vi "Test.vi"() -> ()   [LabVIEW 2014]
uses:
  <vilib>/Utility/file.llb/Read From Spreadsheet File (DBL).vi
  <vilib>/imath/engines/lvmath2/RunTimeEngine/ArithmeticOperatorToken/NIMS_ArithmeticOperator_minus.vi
  <instcachedir>/0/NIMS_ArithmeticOperator_minus_39C0593E74DA4138ACA2AB742906488D.lvgen/NIMS_ArithmeticOperator_minus_39C0593E74DA4138ACA2AB742906488D_003.vi
  <vilib>/imathl/engines/lvmath/Functions/Error Handling/Create Error.vi
  <vilib>/imath/engines/lvmath2/RunTimeEngine/NodeEndStatement/NIMS_NodeEndStatement_Output.vi
  <instcachedir>/0/NIMS_NodeEndStatement_Output_53EC0D466D134D7ABD903AC30B43404B.lvgen/NIMS_NodeEndStatement_Output_53EC0D466D134D7ABD903AC30B43404B_005.vi
  <vilib>/imath/engines/lvmath2/RunTimeEngine/ErrorHandling/NIMS_Finalize Error.vi
panel:
  out "new points":dbl[][](array[numeric]) format="%0.3f"
  out "Local coordinates":dbl[][](array[numeric]) format="%0.3f"
  out "Ynew":dbl[](array[numeric])
  out "Xnew":dbl[](array[numeric])
  in  "File path for new point":path
  in  "File path for local coordinates":path
  in  "File path for global coordinates":path
  out "Global coordinates":dbl[][](array[numeric]) format="%0.3f"
  out "resY":dbl[](array[numeric])
  out "resX":dbl[](array[numeric])
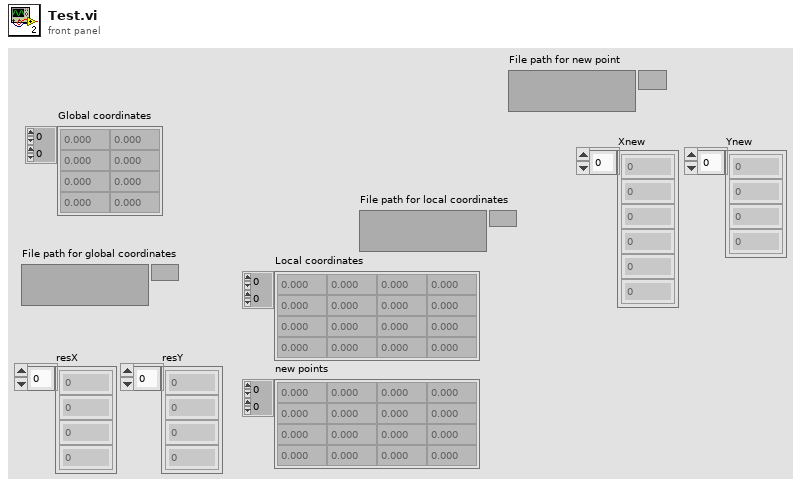
[diagram p1: front panel]
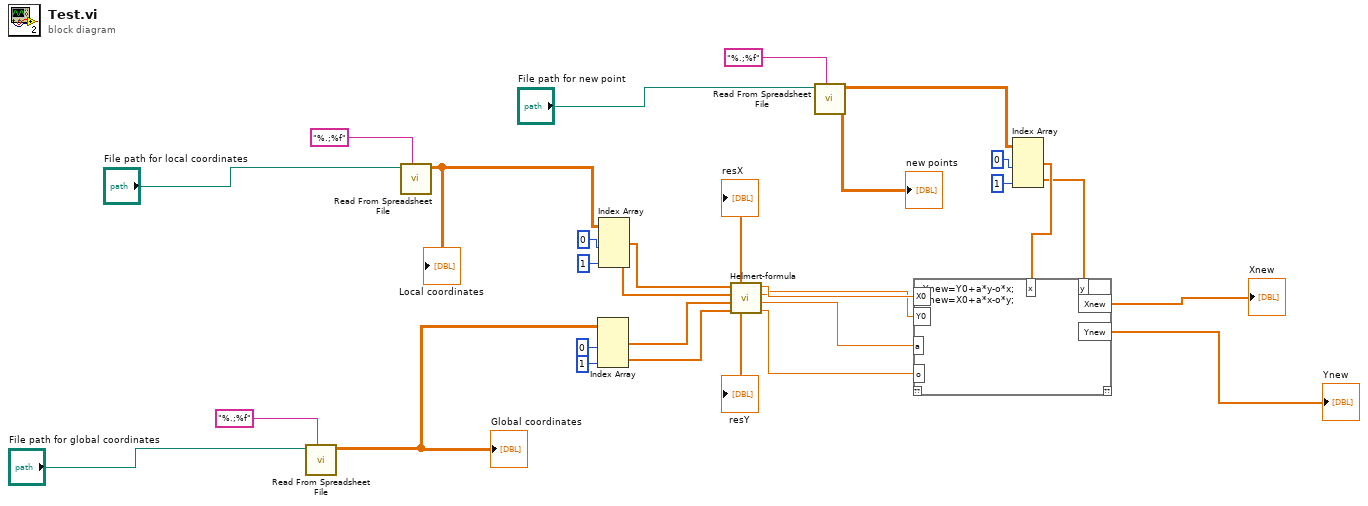
[diagram p0: block diagram]
diagram:
  n1 = call-poly <vilib>:"Read From Spreadsheet File.vi"("format (%.3f)"="%.;%f", "file path (dialog if empty)"="File path for global coordinates") -> ("all rows"=w18:dbl[][])  [unwired: 5 in, 4 out]
  "Global coordinates" <- w18
  n2 = call-poly <vilib>:"Read From Spreadsheet File.vi"("format (%.3f)"="%.;%f", "file path (dialog if empty)"="File path for local coordinates") -> ("all rows"=w15:dbl[][])  [unwired: 5 in, 4 out]
  "Local coordinates" <- w15
  n3 = Index Array(array=w18, index (col) #1=0 ("disabled index (col)"), index (col) #2=1 ("index (col)")) -> (element #1=w24:dbl[], element #2=w23:dbl[])  [unwired: 2 in]
  n4 = Index Array(array=w15, index (col) #1=0 ("index (row)"), index (col) #2=1 ("disabled index (col)")) -> (element #1=w26:dbl[], element #2=w25:dbl[])  [unwired: 2 in]
  n5 = call "Helmert-formula.vi"("Y"=w23, "X"=w24, "y"=w25, "x"=w26) -> ("o"=w14:dbl, "a"=w13:dbl, "Y0"=w11:dbl, "X0"=w12:dbl, "resY"=→"resY":dbl[], "resX"=→"resX":dbl[])  [unwired: 2 in]
  n6 = call-poly <vilib>:"Read From Spreadsheet File.vi"("format (%.3f)"="%.;%f", "file path (dialog if empty)"="File path for new point") -> ("all rows"=w7:dbl[][])  [unwired: 5 in, 4 out]
  "new points" <- w7
  n7 = Index Array(array=w7, index (col) #1=0 ("index (row)"), index (col) #2=1 ("disabled index (col)")) -> (element #1=w6:dbl[], element #2=w5:dbl[])  [unwired: 2 in]
  n8 = mathscript code="Ynew=Y0+a*y-o*x;\nXnew=X0+a*x-o*y;"("X0"=w12, "Y0"=w11, "a"=w13, "o"=w14, "x"=w6, "y"=w5) -> ("Xnew"=→"Xnew":dbl[], "Ynew"=→"Ynew":dbl[])  [unwired: 1 in, 1 out]
